vi "TabControl.vi"(8 "Pages":refnum<vi>[](array[refnum]), 10 "Boolean":bool, 11 "error in (no error)":errorcluster) -> (0 "error out":errorcluster)   [LabVIEW 2013]
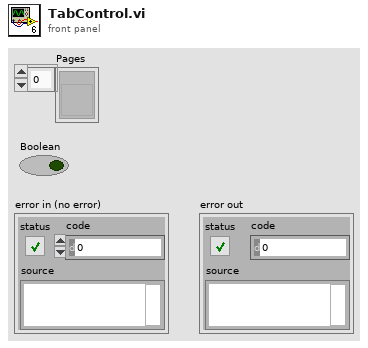
[diagram p1: front panel]
types:
  T1 = enum32{"Page Enabled", "Page Disabled", "Page Disabled & Grayed"}
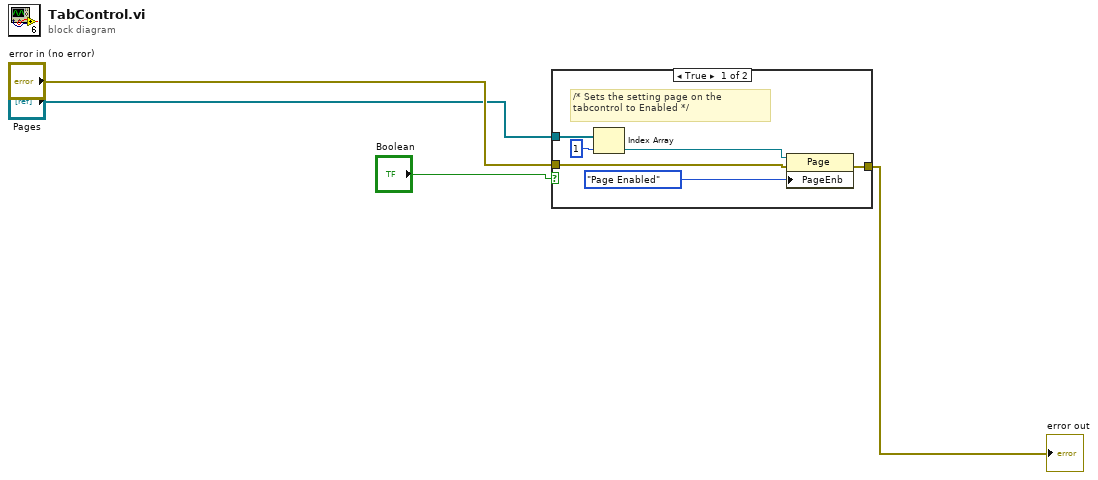
[diagram p0: block diagram]
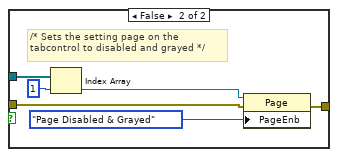
[diagram p2: hidden frame]
diagram:
  n1 = case shown="True" "Boolean" {
    tunnel: "Pages" -> [w9 w15]
    tunnel: "error in (no error)" -> [w6 w12]
    tunnel: [w5 w11] -> w4
    frame True {
      # "/* Sets the setting page on the tabcontrol to Enabled */"
      n2 = Index Array(array=w9, index=1) -> (element=w7:refnum<vi>)
      n3 = property class="Page"(reference=w7, error in=w6, "PageEnb"=T1."Page Enabled" ("Page Enabled State")) -> (error out=w5:errorcluster)  [unwired: 1 out]
    }
    frame False {
      # "/* Sets the setting page on the tabcontrol to disabled and grayed */"
      n4 = Index Array(array=w15, index=1) -> (element=w13:refnum<vi>)
      n5 = property class="Page"(reference=w13, error in=w12, "PageEnb"=T1."Page Disabled & Grayed" ("Page Enabled State")) -> (error out=w11:errorcluster)  [unwired: 1 out]
    }
  }
  "error out" <- w4
